vi "autonSample.vi"(0 "Auton Array":dbl[][](array[numeric]), 5 "MeasuredHeading":dbl, 9 "EncoderDistance":dbl) -> (4 "Left Drive":dbl(knob) scale=-1.0..1.0, 6 "Right Drive":dbl(knob) scale=-1.0..1.0, 10 "Turret Rotation":dbl, 14 "Feeder motor":dbl, 15 "Shooter motor output":dbl)   [LabVIEW 2011]
uses:
  Robot Global Data.vi
  <vilib>/addons/control/pid/pid.llb/PID (DBL).vi
  <vilib>/addons/control/pid/NI_PID_pid.lvlib
panel:
  out "Tzero":i64
  out "AccumDist":dbl
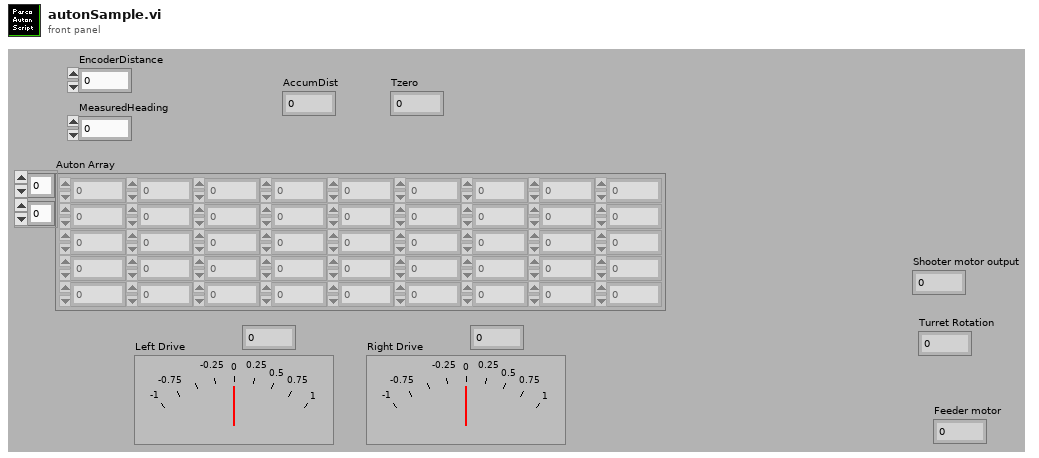
[diagram p1: front panel]
types:
  T1 = cluster{"proportional gain (Kc)":dbl, "integral time (Ti, min)":dbl, "derivative time (Td, min)":dbl}
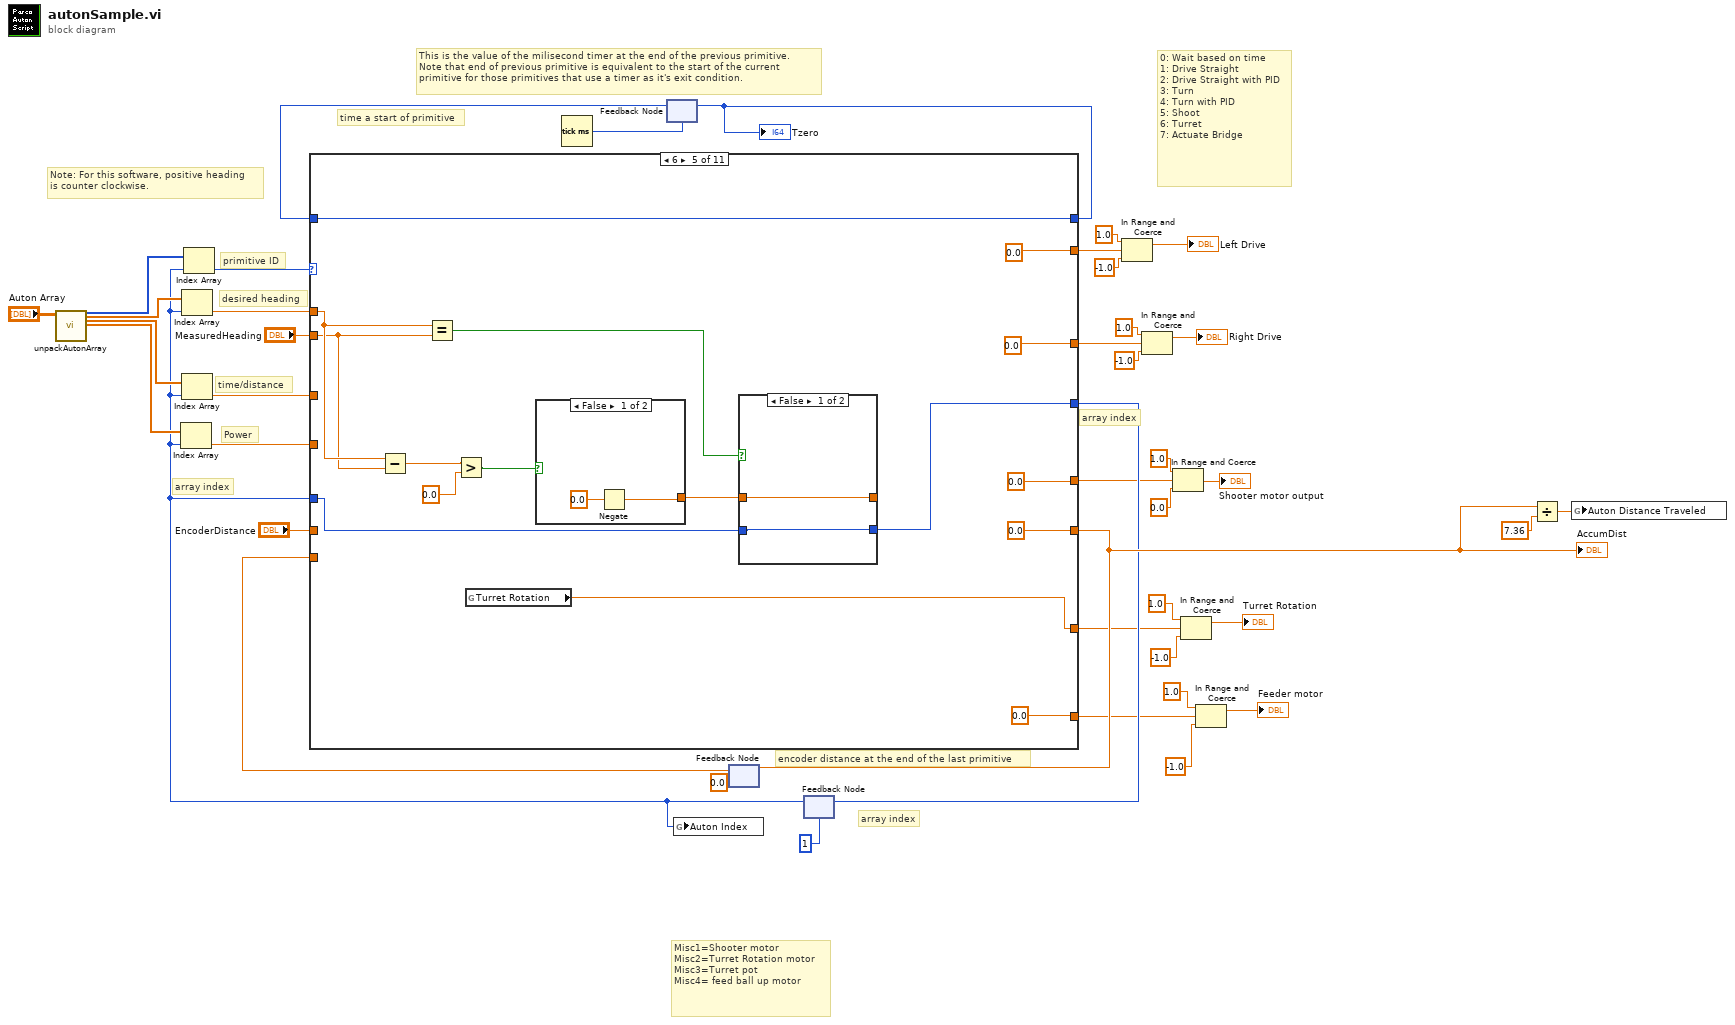
[diagram p0: block diagram]
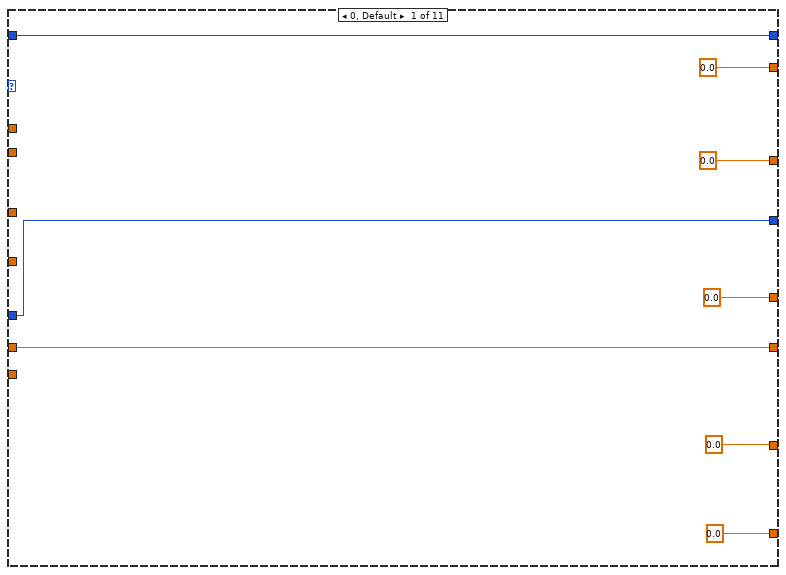
[diagram p2: hidden frame]
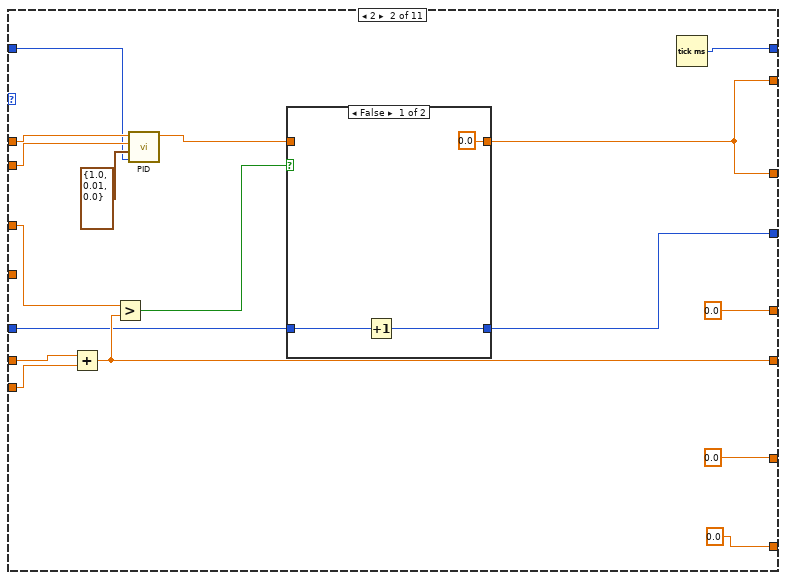
[diagram p3: hidden frame]
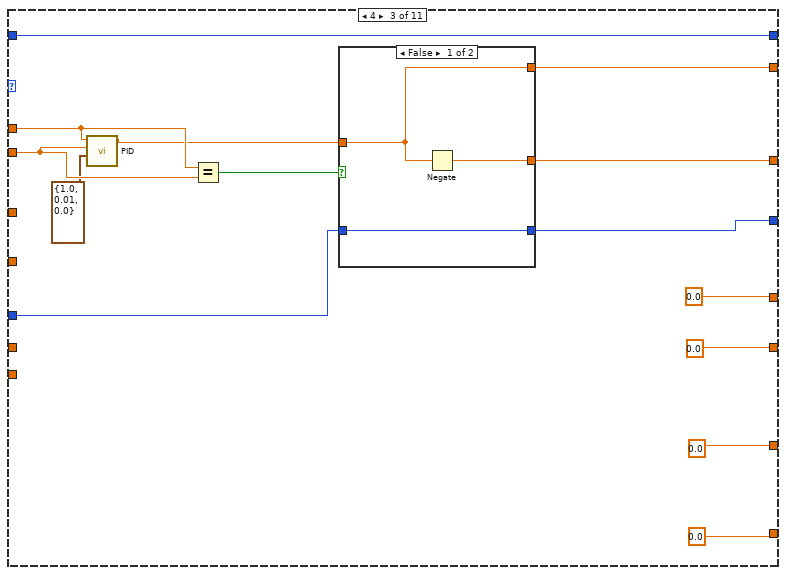
[diagram p5: hidden frame]
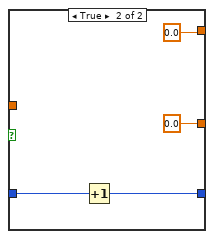
[diagram p6: hidden frame]
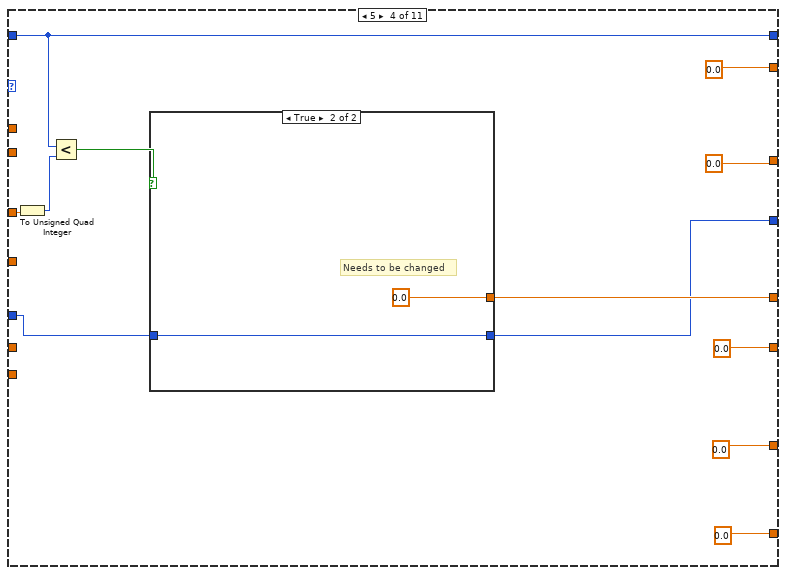
[diagram p7: hidden frame]
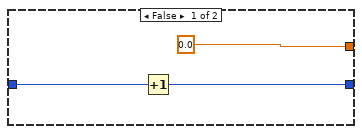
[diagram p8: hidden frame]
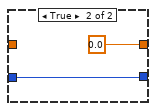
[diagram p9: hidden frame]
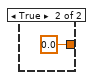
[diagram p10: hidden frame]
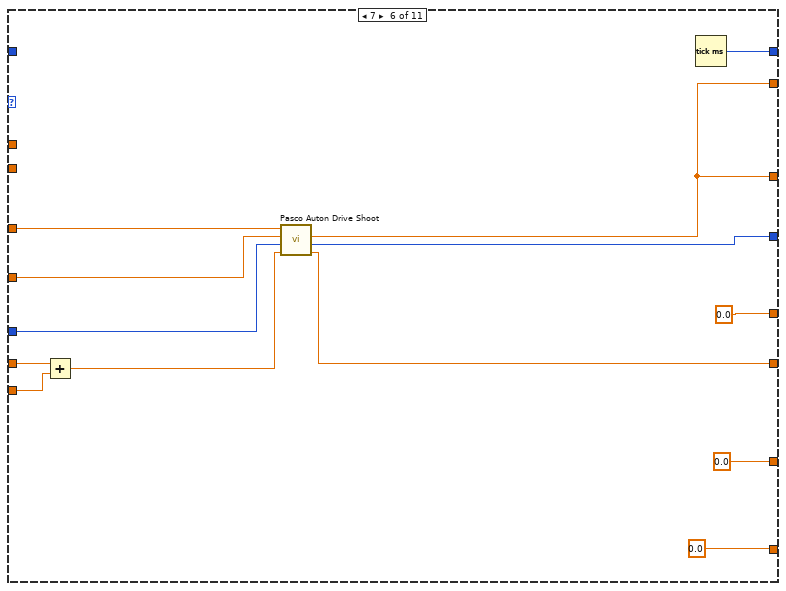
[diagram p11: hidden frame]
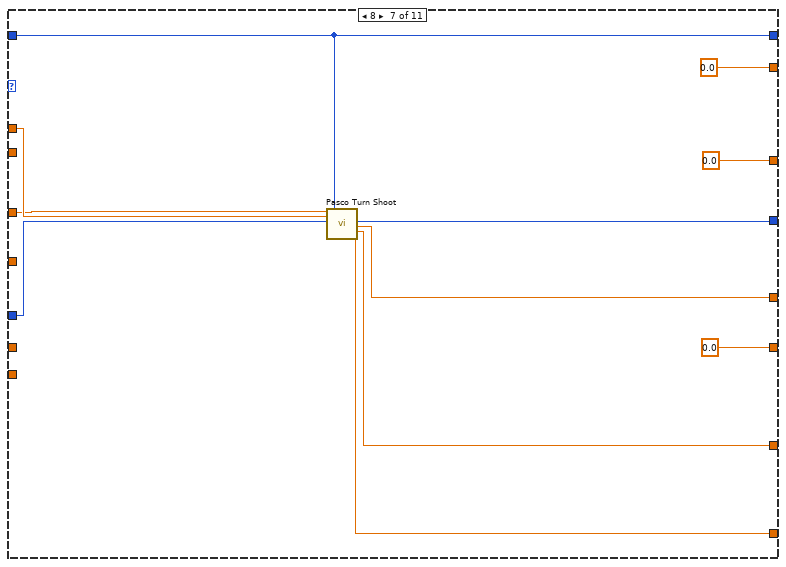
[diagram p12: hidden frame]
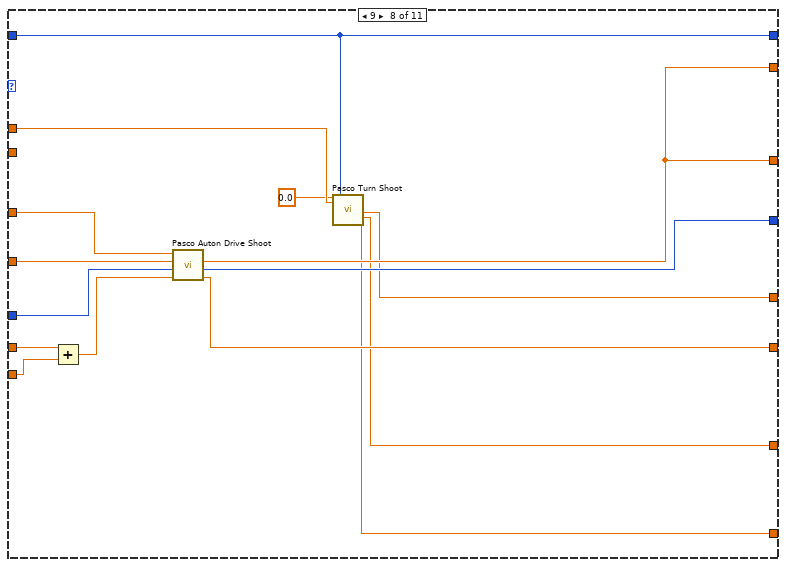
[diagram p13: hidden frame]
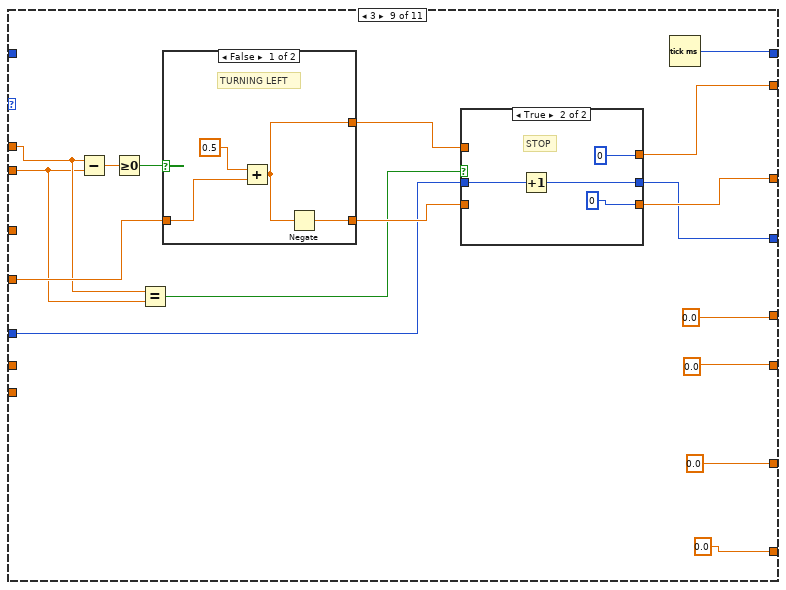
[diagram p14: hidden frame]
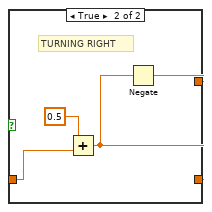
[diagram p16: hidden frame]
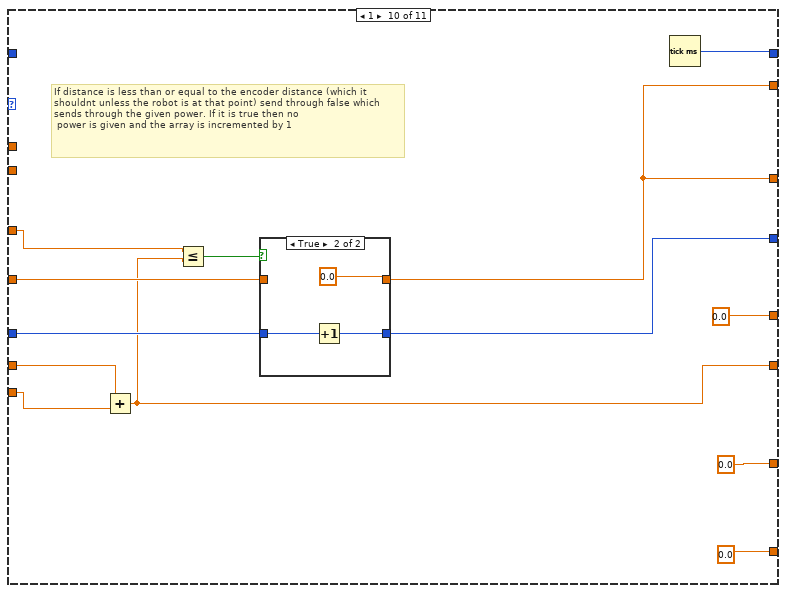
[diagram p17: hidden frame]
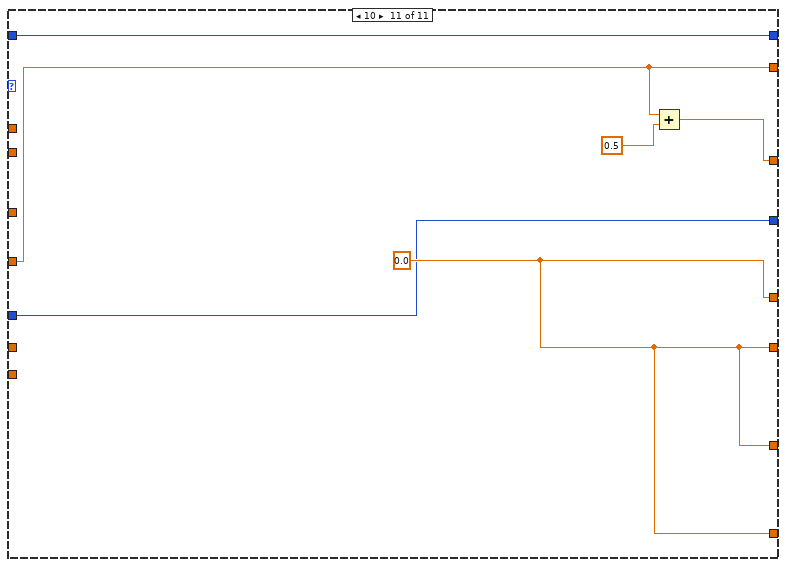
[diagram p19: hidden frame]
diagram:
  # "Misc1=Shooter motor\nMisc2=Turret Rotation motor\nMisc3=Turret pot\nMisc4= feed ball up motor"
  # "0: Wait based on time\n1: Drive Straight\n2: Drive Straight with PID\n3: Turn\n4: Turn with PID\n5: Shoot\n6: Turret\n7: Actuate Bridge"
  # "encoder distance at the end of the last primitive"
  # "Note: For this software, positive heading\nis counter clockwise."
  # "time a start of primitive"
  # "array index"
  # "array index"
  # "This is the value of the milisecond timer at the end of the previous primitive.\nNote that end of previous primitive is equivalent to the start of the current\nprimitive for those primitives that use a timer as it's exit condition."
  # "Power"
  # "array index"
  # "desired heading"
  # "primitive ID"
  # "time/distance"
  n1 = call "unpackAutonArray.vi"("all rows"="Auton Array") -> ("Primitive"=w41:i16[], "Heading"=w23:dbl[], "Distance/Time"=w24:dbl[], "Power"=w21:dbl[])  [unwired: 1 in, 22 out]
  n2 = Tick Count (ms)() -> (millisecond timer value=w35:u32)
  n3 = feedback #1(w35) -> (w39:u32)
  n4 = feedback #2(0.0 ("EncoderDistance")) -> (w20:dbl)
  n5 = feedback #3(1) -> (w2:i32)
  n6 = Index Array(array=w21, index=w2) -> (element=w37:dbl)
  n7 = Index Array(array=w23, index=w2) -> (element=w22:dbl)
  n8 = Index Array(array=w24, index=w2) -> (element=w38:dbl)
  n9 = Index Array(array=w41, index=w2) -> (element=w40:i16)
  n10 = case shown="6" w40 {
    tunnel: [w49 w59 w80 w100 w122 w139 w154 w165 w178 w211 w227] -> w15
    tunnel: w2 -> [w49 w60 w79 w101 w123 w142 w157 w170 w177 w212 w227]
    tunnel: [w46 w67 w86 w95 w121 w135 w155 w160 w184 w210 w226] -> w25
    tunnel: w39 -> [w46 w51 w86 w95 w121 _ w155 w160 _ _ w226]
    tunnel: w38 -> [_ w63 _ w105 _ w146 w151 w172 _ w215 _]
    tunnel: w22 -> [_ w52 w75 _ w126 _ w156 w164 w186 _ _]
    tunnel: [0.0 ("Current Setpoint") w61 w81 0.0 0.0 w140 0.0 w163 w180 w209 w224] -> w33
    tunnel: [0.0 ("Current Setpoint") w61 w82 0.0 0.0 w140 0.0 w163 w183 w209 w223] -> w26
    tunnel: w37 -> [_ _ _ _ _ w141 _ w171 w188 w213 w224]
    tunnel: "EncoderDistance" -> [w50 w66 _ _ _ w145 _ w169 _ w217 _]
    tunnel: "MeasuredHeading" -> [_ w53 w76 _ w112 _ _ _ w185 _ _]
    tunnel: [w50 w64 0.0 0.0 0.0 w138 0.0 w166 0.0 w206 w228] -> w17
    tunnel: w20 -> [_ w65 _ _ _ w144 _ w168 _ w216 _]
    tunnel: [0.0 0.0 0.0 w102 0.0 0.0 ("Misc1  OUT") w153 w162 0.0 0.0 w228] -> w11
    tunnel: [0.0 0.0 0.0 0.0 w111 0.0 ("Misc1  OUT") w152 w161 0.0 0.0 w228] -> w7
    tunnel: [0.0 0.0 0.0 0.0 0.0 0.0 w147 w158 0.0 0.0 w228] -> w3
    frame 0, Default {
    }
    frame 2 {
      n11 = Add(x=w66, y=w65) -> (x+y=w64:dbl)
      n12 = Greater?(x=w63, y=w64) -> (0:w62:bool)
      n13 = call-poly <vilib>:"PID.vi"("dt (s)"=w51, "PID gains"=T1 {"proportional gain (Kc)"=1.0, "integral time (Ti, min)"=0.01, "derivative time (Td, min)"=0.0}, "process variable"=w53, "setpoint"=w52) -> ("output"=w55:dbl)  [unwired: 6 in, 1 out]
      n14 = case shown="False" w62 {
        tunnel: [0.0 w72] -> w61
        tunnel: w55 -> [_ w72]
        tunnel: w60 -> [w70 w71]
        tunnel: [w69 w71] -> w59
        frame False {
          n15 = Increment(x=w70) -> (x+1=w69:i32)
        }
        frame True {
        }
      }
      n16 = Tick Count (ms)() -> (millisecond timer value=w67:u32)
    }
    frame 4 {
      n17 = call-poly <vilib>:"PID.vi"("PID gains"=T1 {"proportional gain (Kc)"=1.0, "integral time (Ti, min)"=0.01, "derivative time (Td, min)"=0.0}, "process variable"=w76, "setpoint"=w75) -> ("output"=w74:dbl)  [unwired: 7 in, 1 out]
      n18 = Equal?(x=w75, y=w76) -> (x = y?=w78:bool)
      n19 = case shown="False" w78 {
        tunnel: w74 -> [w88 _]
        tunnel: [w89 0.0] -> w82
        tunnel: [w88 0.0] -> w81
        tunnel: [w87 w92] -> w80
        tunnel: w79 -> [w87 w93]
        frame False {
          n20 = Negate(x=w88) -> (-x=w89:dbl)
        }
        frame True {
          n21 = Increment(x=w93) -> (x+1=w92:i32)
        }
      }
    }
    frame 5 {
      n22 = To Unsigned Quad Integer(1:w105) -> (0:w103:u64)
      n23 = Less?(x=w95, y=w103) -> (x < y?=w104:bool)
      n24 = case shown="True" w104 {
        tunnel: [0.0 0.0] -> w102
        tunnel: w101 -> [w107 w110]
        tunnel: [w106 w110] -> w100
        frame False {
          n25 = Increment(x=w107) -> (x+1=w106:i32)
        }
        frame True {
          # "Needs to be changed"
        }
      }
    }
    frame 6 {
      n26 = Subtract(x=w126, y=w112) -> (x-y=w114:dbl)
      n27 = Equal?(x=w126, y=w112) -> (x = y?=w125:bool)
      n28 = Greater?(x=w114, y=0.0) -> (0:w115:bool)
      n29 = global read "Robot Global Data.vi" "Turret Rotation"() -> (w111:dbl)
      n30 = case shown="False" w115 {
        tunnel: [w132 0.0] -> w124
        frame False {
          n31 = Negate(x=0.0) -> (-x=w132:dbl)
        }
        frame True {
        }
      }
      n32 = case shown="False" w125 {
        tunnel: [w128 0.0] -> _
        tunnel: w124 -> [w128 _]
        tunnel: w123 -> [w127 w130]
        tunnel: [w127 w130] -> w122
        frame False {
        }
        frame True {
        }
      }
    }
    frame 7 {
      n33 = Add(x=w145, y=w144) -> (x+y=w143:dbl)
      n34 = call "Pasco Auton Drive Shoot.vi"("Encoder total"=w143, "Array"=w142, "Power"=w141, "time/distance"=w146) -> ("Encoder total"=w138:dbl, "Array Out"=w139:i32, "Power"=w140:dbl)  [unwired: 5 in]
      n35 = Tick Count (ms)() -> (millisecond timer value=w135:u32)
    }
    frame 8 {
      n36 = call "Pasco Turn Shoot.vi"("time/distance"=w151, "desired heading"=w156, "array index"=w157, "primitive time"=w155) -> ("array index"=w154:i32, "Misc1  OUT"=w153:dbl, "Misc2 OUT"=w152:dbl, "Misc4 OUT"=w147:dbl)  [unwired: 12 in]
    }
    frame 9 {
      n37 = Add(x=w169, y=w168) -> (x+y=w167:dbl)
      n38 = call "Pasco Auton Drive Shoot.vi"("Encoder total"=w167, "Array"=w170, "Power"=w171, "time/distance"=w172) -> ("Encoder total"=w166:dbl, "Array Out"=w165:i32, "Power"=w163:dbl)  [unwired: 5 in]
      n39 = call "Pasco Turn Shoot.vi"("time/distance"=0.0, "desired heading"=w164, "primitive time"=w160) -> ("Misc1  OUT"=w162:dbl, "Misc2 OUT"=w161:dbl, "Misc4 OUT"=w158:dbl)  [unwired: 13 in, 1 out]
    }
    frame 3 {
      n40 = Subtract(x=w186, y=w185) -> (x-y=w189:dbl)
      n41 = Greater Or Equal To 0?(x=w189) -> (x >= 0?=w187:bool)
      n42 = Equal?(x=w186, y=w185) -> (x = y?=w179:bool)
      n43 = case shown="False" w187 {
        tunnel: w188 -> [w199 w201]
        tunnel: [w197 w203] -> w181
        tunnel: [w198 w202] -> w182
        frame False {
          # "TURNING LEFT"
          n44 = Add(x=0.5, y=w199) -> (x+y=w197:dbl)
          n45 = Negate(x=w197) -> (-x=w198:dbl)
        }
        frame True {
          # "TURNING RIGHT"
          n46 = Add(x=0.5, y=w201) -> (x+y=w202:dbl)
          n47 = Negate(x=w202) -> (-x=w203:dbl)
        }
      }
      n48 = case shown="True" w179 {
        tunnel: w177 -> [w192 w196]
        tunnel: [w192 w195] -> w178
        tunnel: [w191 0] -> w183
        tunnel: w182 -> [w191 _]
        tunnel: [w190 0] -> w180
        tunnel: w181 -> [w190 _]
        frame False {
          # "DRIVE"
        }
        frame True {
          # "STOP"
          n49 = Increment(x=w196) -> (x+1=w195:i32)
        }
      }
      n50 = Tick Count (ms)() -> (millisecond timer value=w184:u32)
    }
    frame 1 {
      # "If distance is less than or equal to the encoder distance (which it shouldnt unless the robot is at that point) send through false which sends through the given power. If it is true then no\n power is given and the array is incremented by 1"
      n51 = Add(x=w217, y=w216) -> (x+y=w206:dbl)
      n52 = Less Or Equal?(x=w215, y=w206) -> (x <= y?=w214:bool)
      n53 = case shown="True" w214 {
        tunnel: [w219 0.0] -> w209
        tunnel: w213 -> [w219 _]
        tunnel: w212 -> [w218 w221]
        tunnel: [w218 w220] -> w211
        frame False {
        }
        frame True {
          n54 = Increment(x=w221) -> (x+1=w220:i32)
        }
      }
      n55 = Tick Count (ms)() -> (millisecond timer value=w210:u32)
    }
    frame 10 {
      w228 = 0.0
      n56 = Add(x=w224, y=0.5 ("x+y")) -> (x+y=w223:dbl)
    }
  }
  "AccumDist" <- w17
  "Tzero" <- w25
  n57 = feedback-in #1(w25) -> ()
  n58 = global write "Robot Global Data.vi" "Auton Index"(w2) -> ()
  n59 = feedback-in #2(w17) -> ()
  n60 = feedback-in #3(w15) -> ()
  n61 = In Range and Coerce(upper limit=1.0, x=w33, lower limit=-1.0) -> (coerced(x)=→"Left Drive":dbl)  [unwired: 1 out]
  n62 = In Range and Coerce(upper limit=1.0, x=w26, lower limit=-1.0) -> (coerced(x)=→"Right Drive":dbl)  [unwired: 1 out]
  n63 = In Range and Coerce(upper limit=1.0, x=w11, lower limit=0.0) -> (coerced(x)=→"Shooter motor output":dbl)  [unwired: 1 out]
  n64 = In Range and Coerce(upper limit=1.0, x=w7, lower limit=-1.0) -> (coerced(x)=→"Turret Rotation":dbl)  [unwired: 1 out]
  n65 = In Range and Coerce(upper limit=1.0, x=w3, lower limit=-1.0) -> (coerced(x)=→"Feeder motor":dbl)  [unwired: 1 out]
  n66 = Divide(x=w17, y=7.36) -> (x/y=w1:dbl)
  n67 = global write "Robot Global Data.vi" "Auton Distance Traveled"(w1) -> ()
